vi "testIsQueueTcpClientFromDdsFull.vi"(8 "error in (no error)":errorcluster) -> (0 "error out":errorcluster)   [LabVIEW 2018]
doc: "Test the IsQueueTcpClientFull.vi with queueFromDds option."
uses:
  src/TcpServer/TcpServer.lvclass
  src/TcpServer/configServerTypeDef.ctl
  src/TcpServerTel/typedef/enqueueOptionsTypeDef.ctl
  src/TcpServer/TcpServer.lvclass/TcpServer.ctl
  src/TcpServerTel/TcpServerTel.lvclass/TcpServerTel.ctl
  <vilib>/addons/_JKI Toolkits/Caraya/classes/Assert/Assert False.vi
  <vilib>/addons/_JKI Toolkits/Caraya/classes/Assert/Assert True.vi
  src/TcpServerTel/TcpServerTel.lvclass
  <vilib>/addons/_JKI Toolkits/Caraya/classes/Test/Test.lvclass
  <vilib>/addons/_JKI Toolkits/Caraya/classes/Assert/Assert.lvclass
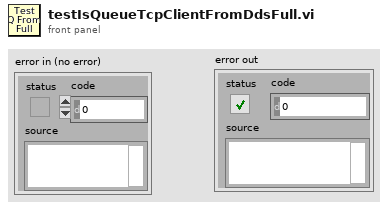
[diagram p1: front panel]
types:
  T1 = enum16{"queueTcpClientFromDds", "queueTcpClient"}
  T2 = typedef "TcpServer.lvclass/configServerTypeDef.ctl" = cluster{"cmdServerPort":u16, "telServerPort":u16, "serverTimeout (ms)":i32, "serverBytesToRead":i32, "maxSizeQueueTcpClientFromDds":i32, "EnqueueOptions":T3, "timeoutQueueTcpClientFromDds (ms)":i32, "maxSizeQueueTcpClient":i32, "timeoutInMs":i32}
  T3 = typedef "TcpServerTel.lvclass/enqueueOptionsTypeDef.ctl" = enum16{"lossy enqueue", "normal enqueue"}
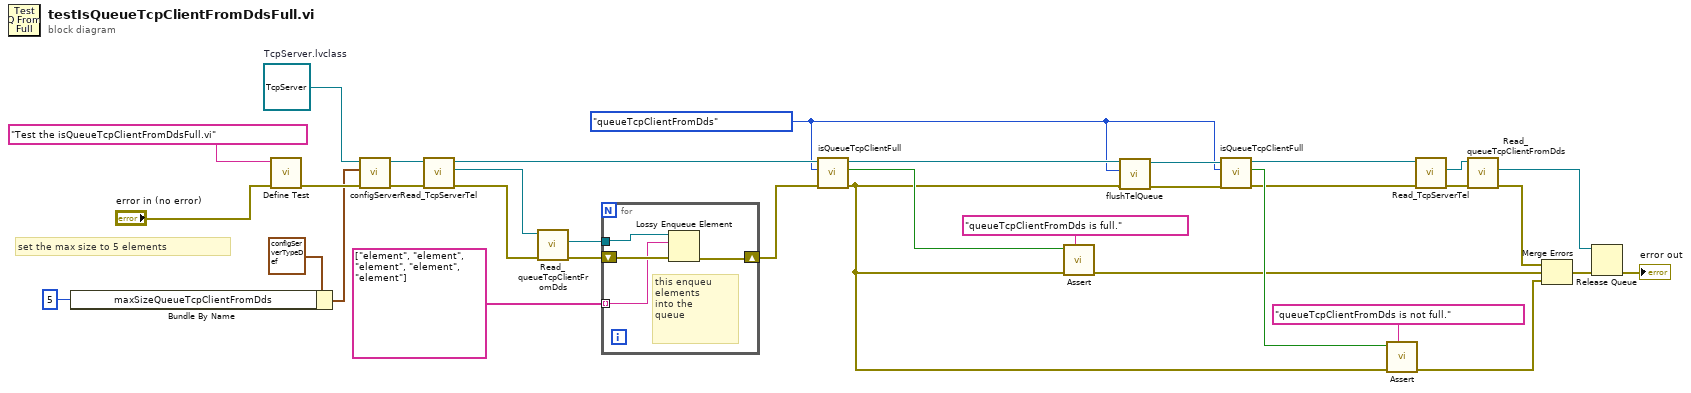
[diagram p0: block diagram]
diagram:
  w1 = T1."queueTcpClientFromDds" ("queueName")
  w24 = refnum<class "TcpServer.lvclass"> refnum  # TcpServer.lvclass
  # "set the max size to 5 elements"
  n1 = Bundle By Name(cluster=T2 {"cmdServerPort"=8888, "telServerPort"=8889, "serverTimeout (ms)"=100, "serverBytesToRead"=32768, "maxSizeQueueTcpClientFromDds"=1000, "EnqueueOptions"=enum."lossy enqueue", "timeoutQueueTcpClientFromDds (ms)"=50, "maxSizeQueueTcpClient"=1000, "timeoutInMs"=100} ("ServerConfiguration"), "maxSizeQueueTcpClientFromDds"=5 ("telQueueServerMaxSize")) -> (w3:T2)
  n2 = call <vilib>:"Define Test.vi"("error in (no error)"="error in (no error)", "Label (VI Title)"="Test the isQueueTcpClientFromDdsFull.vi") -> ("error out"=w23:errorcluster)  [unwired: 9 in]
  n3 = call "configServer.vi"("error in (no error)"=w23, "ServerConfiguration"=w3, "tcpServer in"=w24) -> ("error out"=w11:errorcluster, "tcpServer out"=w12:refnum<class "TcpServer.lvclass">)  [unwired: 7 in]
  n4 = call "Read_TcpServerTel.vi"("error in (no error)"=w11, "TcpServer in"=w12) -> ("error out"=w10:errorcluster, "TcpServerTel.lvclass"=w9:refnum<class "TcpServerTel.lvclass">, "TcpServer out"=w8:refnum<class "TcpServer.lvclass">)  [unwired: 7 in]
  n5 = call "Read_queueTcpClientFromDds.vi"("error in (no error)"=w10, "TcpServerTel in"=w9) -> ("error out"=w14:errorcluster, "queueTcpClientFromDds"=w13:refnum<queue>)  [unwired: 7 in, 1 out]
  n6 = for {
    shift-right: [w38] -> w7
    shift-left: w14 -> [w39]
    tunnel: string[] ["element", "element", "element", "element", "element"] -> [w36] mode=indexing
    tunnel: w13 -> [w37]
    # "this enqueu\nelements\ninto the\nqueue"
    n7 = Lossy Enqueue Element(queue=w37, element=w36, error in (no error)=w39) -> (error out=w38:errorcluster)  [unwired: 3 out]
  }
  n8 = call "isQueueTcpClientFull.vi"("error in (no error)"=w7, "queueName"=w1, "tcpServer in"=w8) -> ("error out"=w5:errorcluster, "queueFull"=w30:bool, "tcpServer out"=w22:refnum<class "TcpServer.lvclass">)  [unwired: 6 in]
  n9 = call-poly <vilib>:"Assert.vi"("Label"="queueTcpClientFromDds is full.", "error in (no error)"=w5, "True?"=w30) -> ("error out"=w17:errorcluster)  [unwired: 8 in]
  n10 = call "flushTelQueue.vi"("error in (no error)"=w5, "queueName"=w1, "TcpServer in"=w22) -> ("error out"=w4:errorcluster, "TcpServer out"=w6:refnum<class "TcpServer.lvclass">)  [unwired: 6 in, 1 out]
  n11 = call "isQueueTcpClientFull.vi"("error in (no error)"=w4, "queueName"=w1, "tcpServer in"=w6) -> ("error out"=w18:errorcluster, "queueFull"=w20:bool, "tcpServer out"=w19:refnum<class "TcpServer.lvclass">)  [unwired: 6 in]
  n12 = call-poly <vilib>:"Assert.vi"("Label"="queueTcpClientFromDds is not full.", "error in (no error)"=w5, "False?"=w20) -> ("error out"=w16:errorcluster)  [unwired: 8 in]
  n13 = call "Read_TcpServerTel.vi"("error in (no error)"=w18, "TcpServer in"=w19) -> ("error out"=w29:errorcluster, "TcpServerTel.lvclass"=w28:refnum<class "TcpServerTel.lvclass">)  [unwired: 7 in, 1 out]
  n14 = call "Read_queueTcpClientFromDds.vi"("error in (no error)"=w29, "TcpServerTel in"=w28) -> ("error out"=w26:errorcluster, "queueTcpClientFromDds"=w27:refnum<queue>)  [unwired: 7 in, 1 out]
  n15 = Merge Errors(w26, w17, w16) -> (w31:errorcluster)
  n16 = Release Queue(queue=w27, error in (no error)=w31) -> (error out=→"error out":errorcluster)  [unwired: 1 in, 2 out]
